vi "removeDeviceListBox.vi"(8 "error in (no error)":errorcluster, 10 "index":i32, 11 "reference":refnum<vi>) -> (0 "error out":errorcluster, 3 "reference out":refnum<vi>)   [LabVIEW 2010]
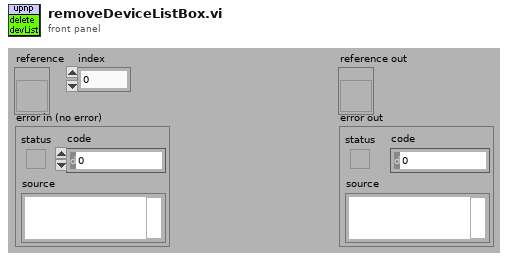
[diagram p1: front panel]
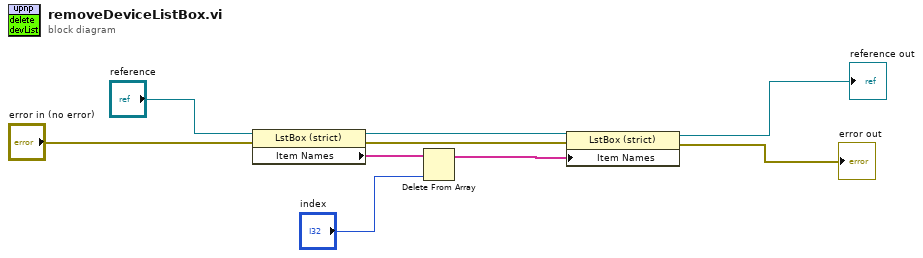
[diagram p0: block diagram]
diagram:
  n1 = property class="LstBox (strict)"(reference="reference", error in="error in (no error)") -> (reference out=w4:refnum<vi>, error out=w3:errorcluster, "Item Names"=w7:string[])
  n2 = Delete From Array(array=w7, index="index") -> (array with subset deleted=w5:string[])  [unwired: 1 in, 1 out]
  n3 = property class="LstBox (strict)"(reference=w4, error in=w3, "Item Names"=w5) -> (reference out=→"reference out":refnum<vi>, error out=→"error out":errorcluster)
